vi "GENser Config Output On-Off.vi"(7 "GEN Addr":i16=-1, 8 "error":errorcluster, 9 "Settle (0 mS)":u32, 10 "Output ON":bool, 11 "VISA":refnum<visa-resource-name>) -> (0 "error out":errorcluster, 3 "VISA out":refnum<visa-resource-name>)   [LabVIEW 2017]
doc: "This VI sets the power supply output ON or OFF. No other settings change.\nIf \"Output ON\" is set FALSE, the output will be turned OFF.\n\nThis VI will wait for \"Settle\" milliseconds after setting the output. If unwired, there will be no delay\n\nNote: Some power supply faults will prevent the output from being turned ON. In this case, an error will be returned."
panel:
  # "Lambda Genesys \n Serial Port\n  DC Power Supplies"
  # "Set Output ON or OFF"
  # "-1 = no address change"
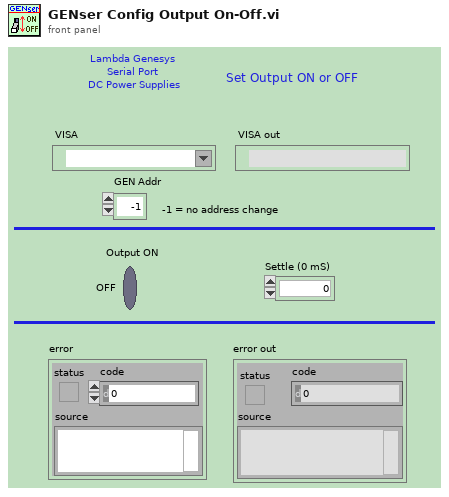
[diagram p1: front panel]
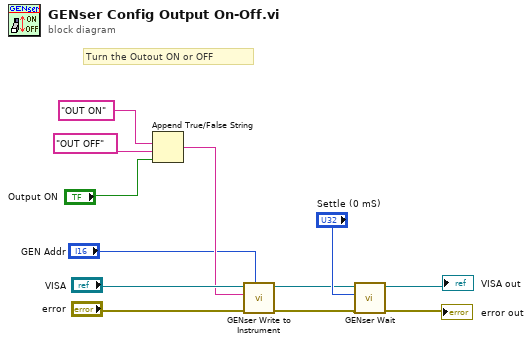
[diagram p0: block diagram]
diagram:
  # "Turn the Outout ON or OFF"
  n1 = Append True/False String(1:"Output ON", 2:"OUT OFF" ("format string"), 3:"OUT ON" ("format string")) -> (0:w4:string)  [unwired: 1 in]
  n2 = call "GENser Write to Instrument.vi"("GEN Addr"="GEN Addr", "error"="error", "Command"=w4, "VISA"="VISA") -> ("error out"=w8:errorcluster, "VISA out"=w7:refnum<visa-resource-name>)  [unwired: 5 in, 1 out]
  n3 = call "GENser Wait.vi"("error"=w8, "Delay (20 mS)"="Settle (0 mS)", "VISA"=w7) -> ("error out"=→"error out":errorcluster, "VISA out"=→"VISA out":refnum<visa-resource-name>)  [unwired: 7 in]
